vi "TEST_AddDocument.vi"() -> ()   [LabVIEW 2020]
uses:
  ProligentResultProcessor/Datawarehouse/Datawarehouse.lvclass
  ProligentResultProcessor/ProductUnit/ProductUnit.lvclass
panel:
  out "error out":errorcluster
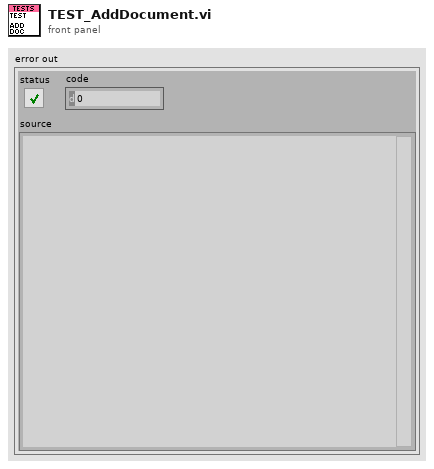
[diagram p1: front panel]
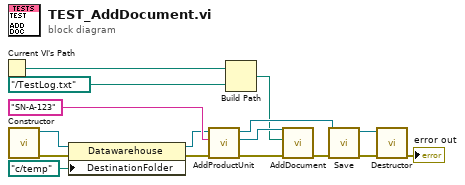
[diagram p0: block diagram]
diagram:
  n1 = Current VI's Path() -> (path=w8:path)
  n2 = call "Constructor.vi"() -> ("error out"=w16:errorcluster, "Datawarehouse"=w3:refnum<class "Datawarehouse.lvclass">)  [unwired: 10 in]
  n3 = property class="Datawarehouse"(reference=w3, error in=w16, "DestinationFolder"=path "c:/temp") -> (reference out=w2:refnum<class "Datawarehouse.lvclass">, error out=w4:errorcluster)
  n4 = call "AddProductUnit.vi"("error in"=w4, "ProductUnitIdentifier"="SN-A-123", "Datawarehouse in"=w2) -> ("error out"=w15:errorcluster, "ProductUnit"=w10:refnum<class "ProductUnit.lvclass">, "Datawarehouse out"=w11:refnum<class "Datawarehouse.lvclass">)  [unwired: 6 in]
  n5 = Build Path(base path=w8, name or relative path=path "../TestLog.txt" ("FilePath")) -> (appended path=w6:path)
  n6 = call "AddDocument.vi"("error in"=w15, "FilePath"=w6, "ProductUnit in"=w10) -> ("error out"=w14:errorcluster)  [unwired: 6 in, 2 out]
  n7 = call "Save.vi"("error in"=w14, "Datawarehouse in"=w11) -> ("error out"=w12:errorcluster, "Datawarehouse out"=w13:refnum<class "Datawarehouse.lvclass">)  [unwired: 8 in]
  n8 = call "Destructor.vi"("error in"=w12, "Datawarehouse"=w13) -> ("error out"=→"error out":errorcluster)  [unwired: 9 in]
